vi "GetSweepConfig.vi"(8 "error in (no error)":errorcluster, 9 "DataGroup":string, 10 "AcqParams":variant, 11 "map in":T2) -> (0 "error out":errorcluster, 1 "OpState":string, 2 "sweep config":T1, 3 "map out":T2)   [LabVIEW 2017, in "EmsaDataEventCreator.lvlib"]
uses:
  <vilib>/addons/InsightCM/Devices/Shared/Emsa/EmsaDataEventCreator/EmsaDataEventCreator.lvlib
  <vilib>/addons/PointValueMap/controls/PointMap.ctl
  <vilib>/addons/InsightCM/Devices/Shared/Emsa/EmsaDataEventCreator/controls/SweepParams.ctl
  <vilib>/addons/PointValueMap/subVIs/Point_Read_string.vi
  <vilib>/addons/PointValueMap/PointValueMap.lvlib
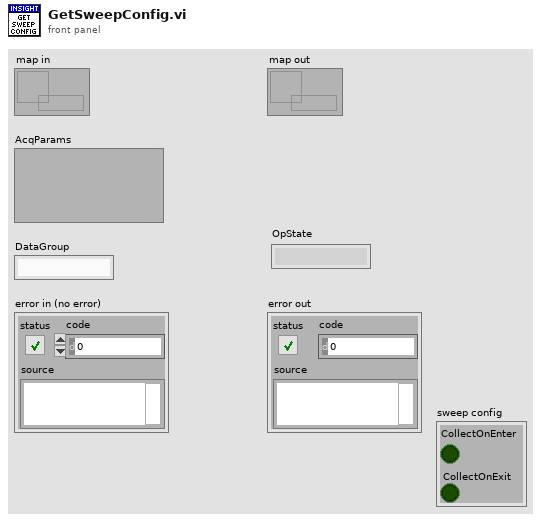
[diagram p1: front panel]
types:
  T1 = typedef "EmsaDataEventCreator.lvlib/SweepParams.ctl" = cluster{"CollectOnEnter":bool, "CollectOnExit":bool}
  T2 = typedef "PointValueMap.lvlib/PointMap.ctl" = refnum<data-value>
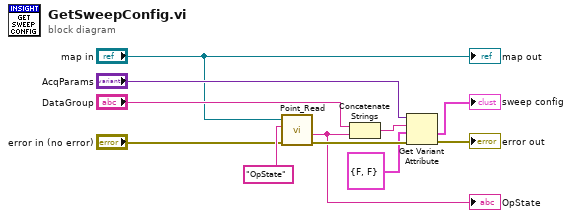
[diagram p0: block diagram]
diagram:
  n1 = call-poly <vilib>:"Point_Read.vi"("Error In"="error in (no error)", "Tag"="OpState", "Map"="map in") -> ("Error Out"=w10:errorcluster, "Value"=w3:string)  [unwired: 3 in, 4 out]
  "OpState" <- w3
  n2 = Concatenate Strings("DataGroup", w3) -> (w11:string)
  n3 = Get Variant Attribute(Variant="AcqParams", name=w11, default value (empty Variant)=T1 {"CollectOnEnter"=FALSE, "CollectOnExit"=FALSE} ("Sweep Params"), error in=w10) -> (value=→"sweep config":T1, error out=→"error out":errorcluster)  [unwired: 2 out]
  "map out" <- "map in"
